vi "Read Many Settings.vi"(0 "Pulse Generator.lvclass in":refnum<class "Pulse Generator.lvclass">, 5 "error in (no error)":errorcluster) -> (10 "Overall Frequency":dbl[unit], 11 "Outputs 1/!1/2/!2":bool[](array[boolean]), 12 "Output Levels.1 High":dbl[unit], 13 "Ch2Width":dbl[unit], 14 "Pulse Generator.lvclass out":refnum<class "Pulse Generator.lvclass">, 15 "Output Levels.1 Low":dbl[unit], 16 "Ch1Width":dbl[unit], 17 "Output Levels.2 High":dbl[unit], 18 "Output Levels.2 Low":dbl[unit], 19 "error out":errorcluster)   [LabVIEW 2017, in "Pulse Generator.lvclass"]
uses:
  Pulse Generator.lvclass
  Pulse Generator.lvclass/Pulse Generator.ctl
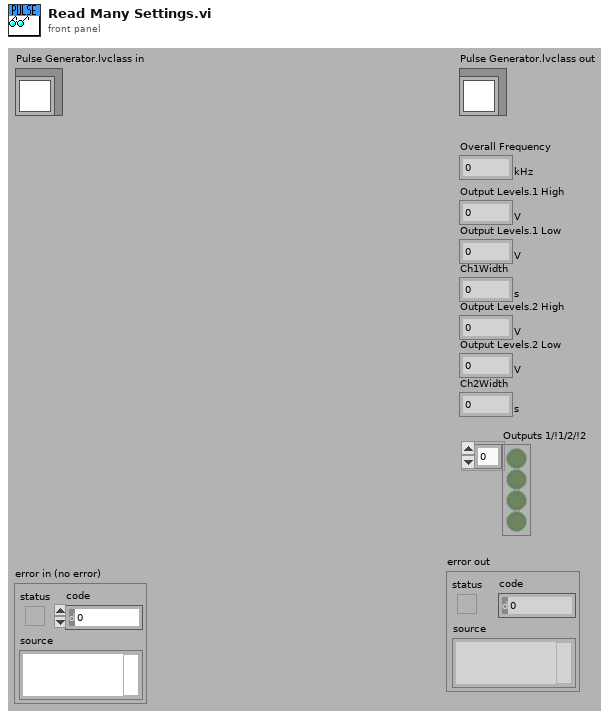
[diagram p1: front panel]
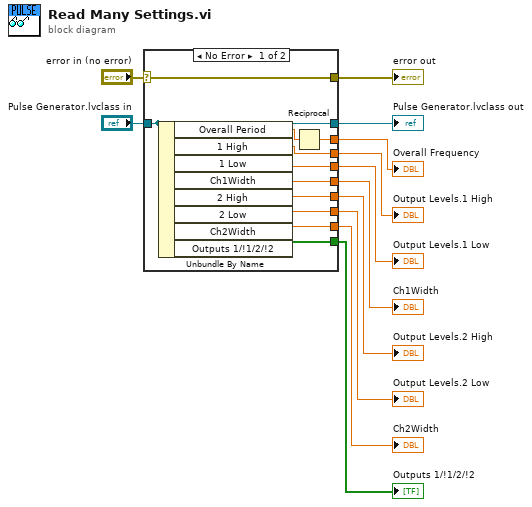
[diagram p0: block diagram]
diagram:
  n1 = case shown="No Error" "error in (no error)" {
    selector: "error in (no error)" -> [w23 w24]
    tunnel: [w23 w24] -> w11
    tunnel: [w22 w25] -> w9
    tunnel: "Pulse Generator.lvclass in" -> [w22 w25]
    tunnel: [w20 _] -> w8
    tunnel: [w19 _] -> w7
    tunnel: [w18 _] -> w6
    tunnel: [w17 _] -> w5
    tunnel: [w16 _] -> w4
    tunnel: [w15 _] -> w3
    tunnel: [w14 _] -> w2
    tunnel: [w13 _] -> w1
    frame No Error {
      n2 = Unbundle By Name(w22) -> ("Overall Period"=w21:dbl[unit], "1 High"=w19:dbl[unit], "1 Low"=w18:dbl[unit], "Ch1Width"=w17:dbl[unit], "2 High"=w16:dbl[unit], "2 Low"=w15:dbl[unit], "Ch2Width"=w14:dbl[unit], "Outputs 1/!1/2/!2"=w13:bool[])
      n3 = Reciprocal(x=w21) -> (1/x=w20:dbl[unit])
    }
    frame Error {
    }
  }
  "error out" <- w11
  "Pulse Generator.lvclass out" <- w9
  "Overall Frequency" <- w8
  "Output Levels.1 High" <- w7
  "Output Levels.1 Low" <- w6
  "Ch1Width" <- w5
  "Output Levels.2 High" <- w4
  "Output Levels.2 Low" <- w3
  "Ch2Width" <- w2
  "Outputs 1/!1/2/!2" <- w1
